vi "相机4图像处理.vi"(6 "生产统计4":T1, 8 "零件型号":string, 9 "工单信息":T2, 10 "自动":bool, 11 "Image Out":T3) -> (0 "生产统计4":T1, 1 "4处理时间":u16, 2 "4结果":bool=TRUE, 3 "Img out":T3(plugin-control))   [LabVIEW 2014]
uses:
  Controls/ProductNum.ctl
  <vilib>/vision/Image Controls.llb/IMAQ Image.ctl
panel:
  in  "显示坐标":cluster{dbl, "Numeric":dbl}[](array[cluster])=[{300.0, "Numeric"=200.0}, {300.0, "Numeric"=400.0}, {300.0, "Numeric"=600.0}, {300.0, "Numeric"=800.0}, {300.0, "Numeric"=1000.0}, {300.0, "Numeric"=1200.0}, {300.0, "Numeric"=1400.0}]
  in  "Img Path":path=path "E:/X-Max总装机3-2019200319/实验图片/4号相机/4.bmp"
  # "%"
  # "%"
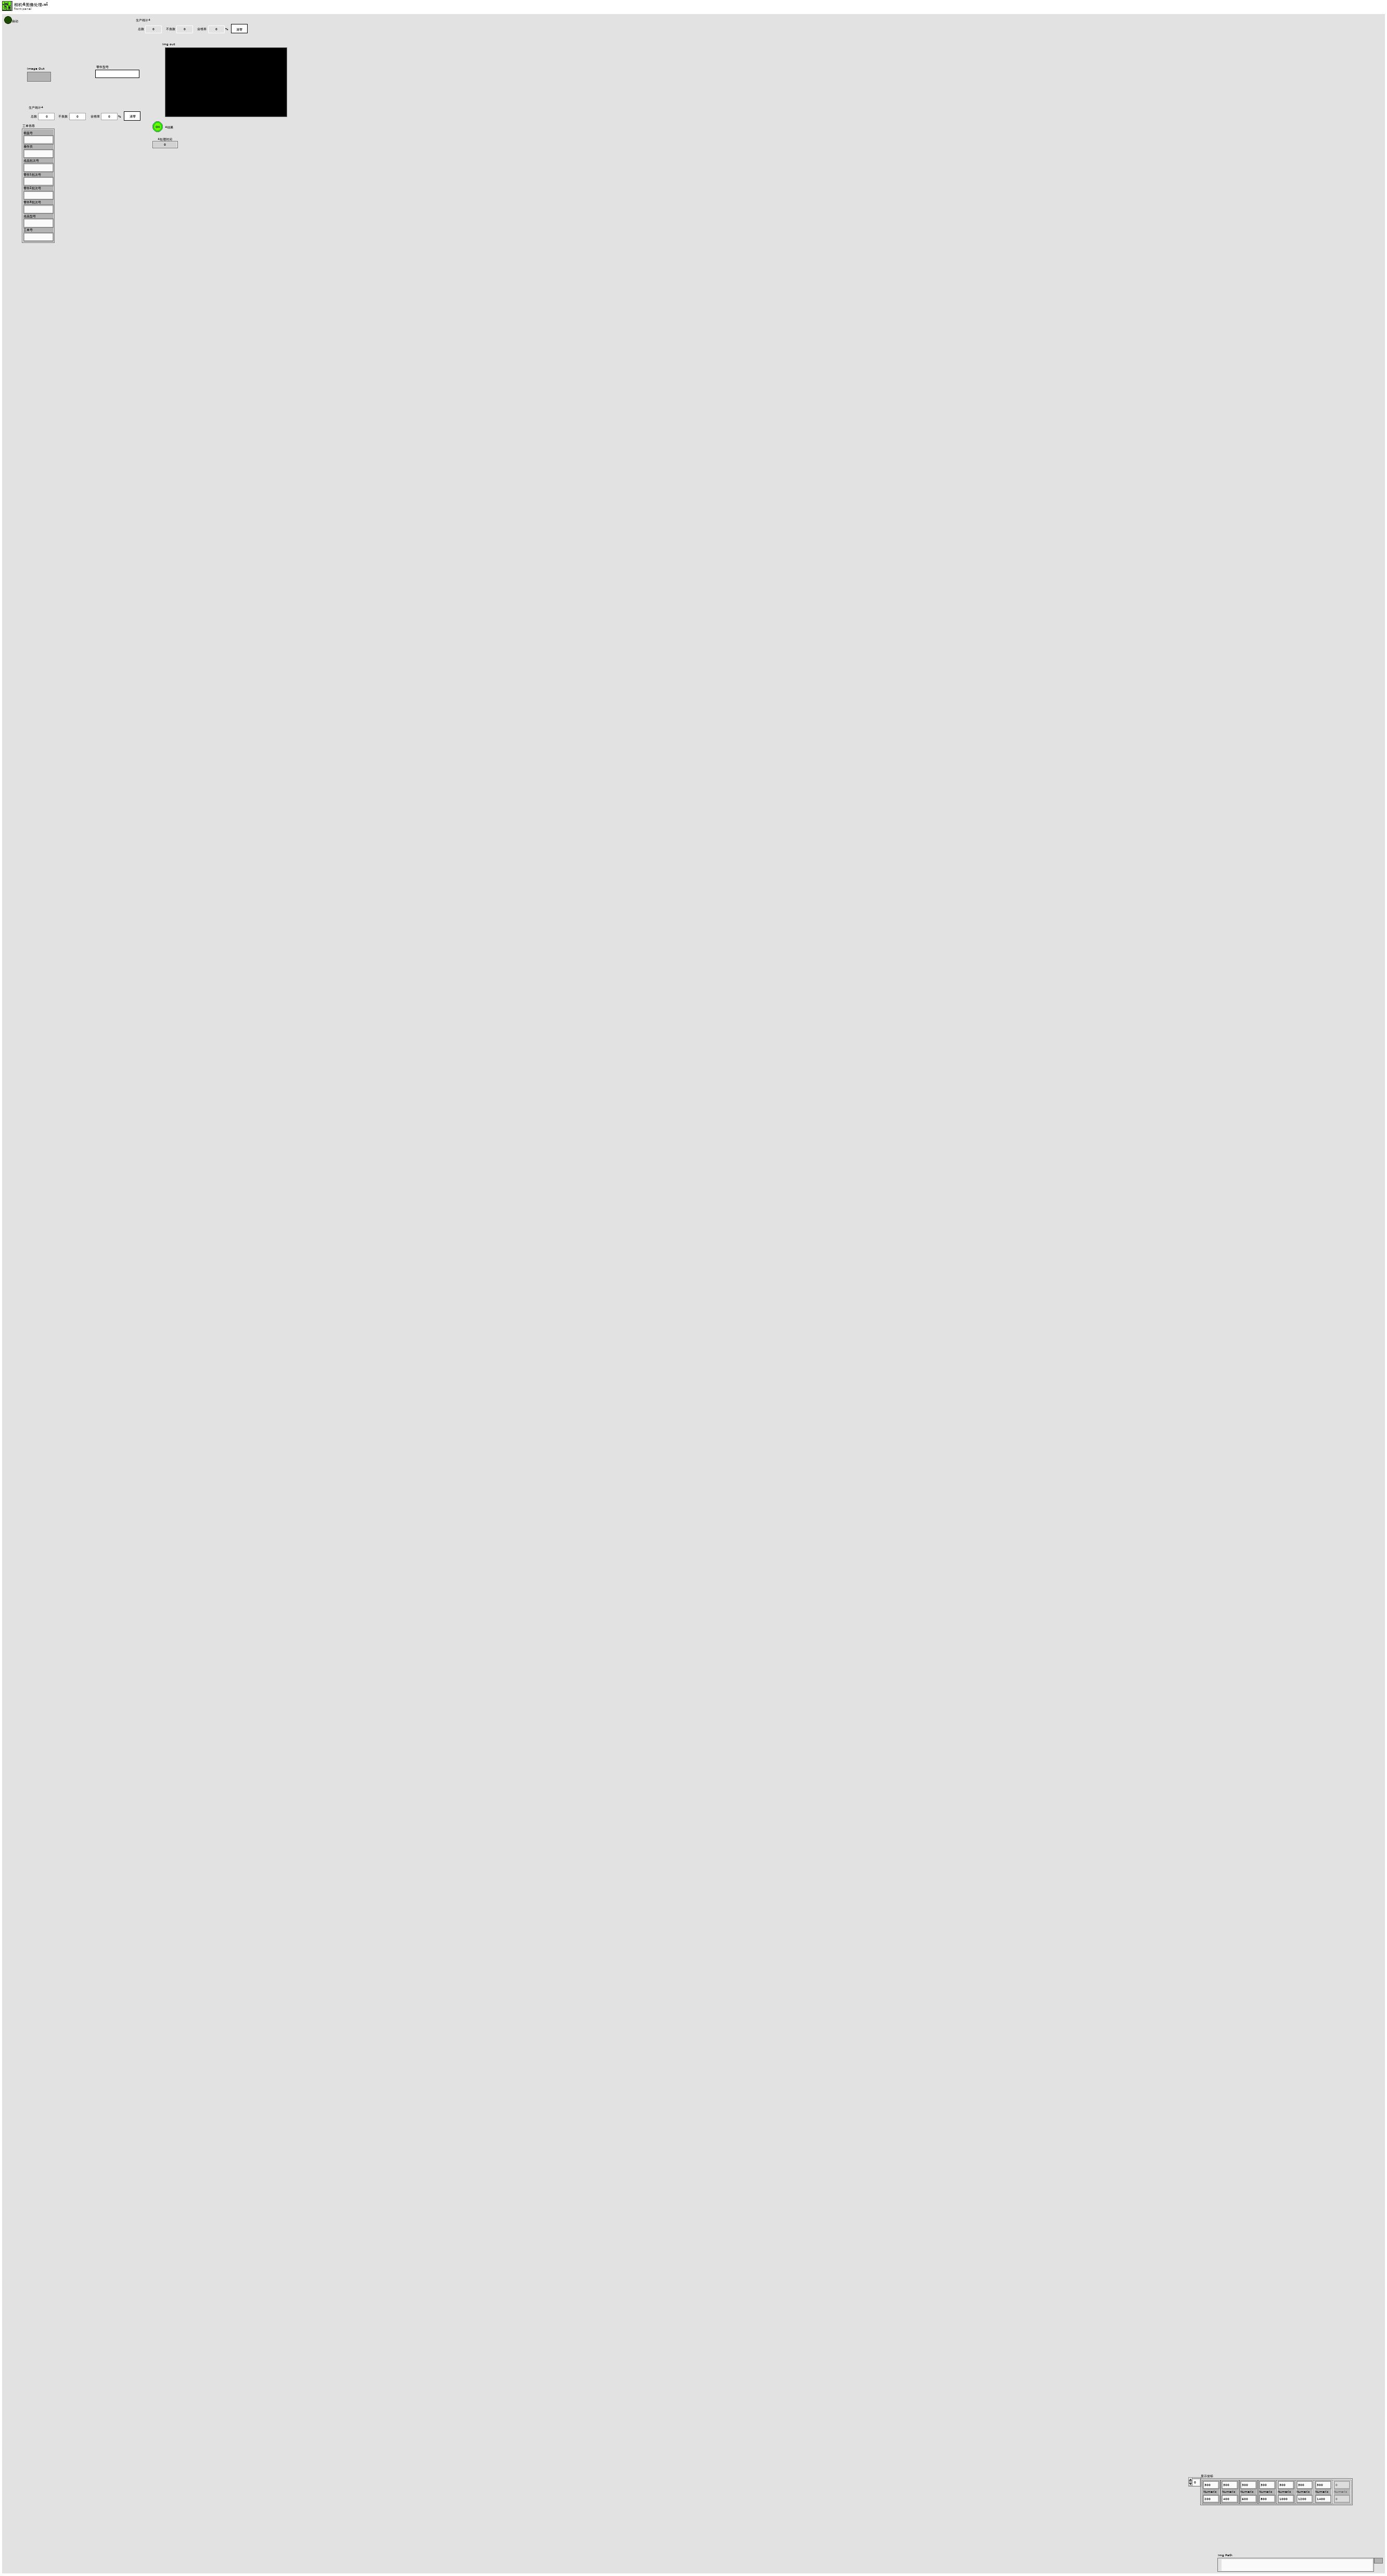
[diagram p1: front panel]
types:
  T1 = typedef "ProductNum.ctl" = cluster{"总数":u64, "不良数":u64, "合格率":dbl, "清零":bool}
  T2 = cluster{"载盘号":string, "操作员":string, "成品批次号":string, "零件1批次号":string, "零件2批次号":string, "零件3批次号":string, "成品型号":string, "工单号":string}
  T3 = typedef "IMAQ Image.ctl" = refnum<image>
  T4 = cluster{"Center (Pixels)":cluster{"X":sgl, "Y":sgl}, "Radius (Pixels)":dbl, "Center (Real-World)":cluster{"X":sgl, "Y":sgl}, "Radius (Real-World)":dbl, "Roundness (Real-World)":dbl, "Average Strength":dbl, "Average SNR (dB)":dbl}
  T5 = typedef "升立德IOAction.ctl" = enum16{"IO卡初始化", "读信号(16bit)", "写信号(16bit)", "写拍照完成信号OFF", "写拍照完成信号ON", "写拍照结果", "GetInfo", "清除目标"}
  T6 = typedef "控件-写数据到PLC Action.ctl" = enum16{"PLC通讯初始化", "PLC通讯初始化2", "读触发信息", "读工单信息", "写工单切换成功", "写入相机1拍照结果", "写入相机2拍照结果", "写入相机3拍照结果", "写入相机4拍照结果", "写入生命信号", "断开连接"}
  T7 = typedef "控件-存档数据和结果.ctl" = cluster{"待写入数据":dbl[], "单个结果":bool[], "总结果":bool, "有效数据":bool}
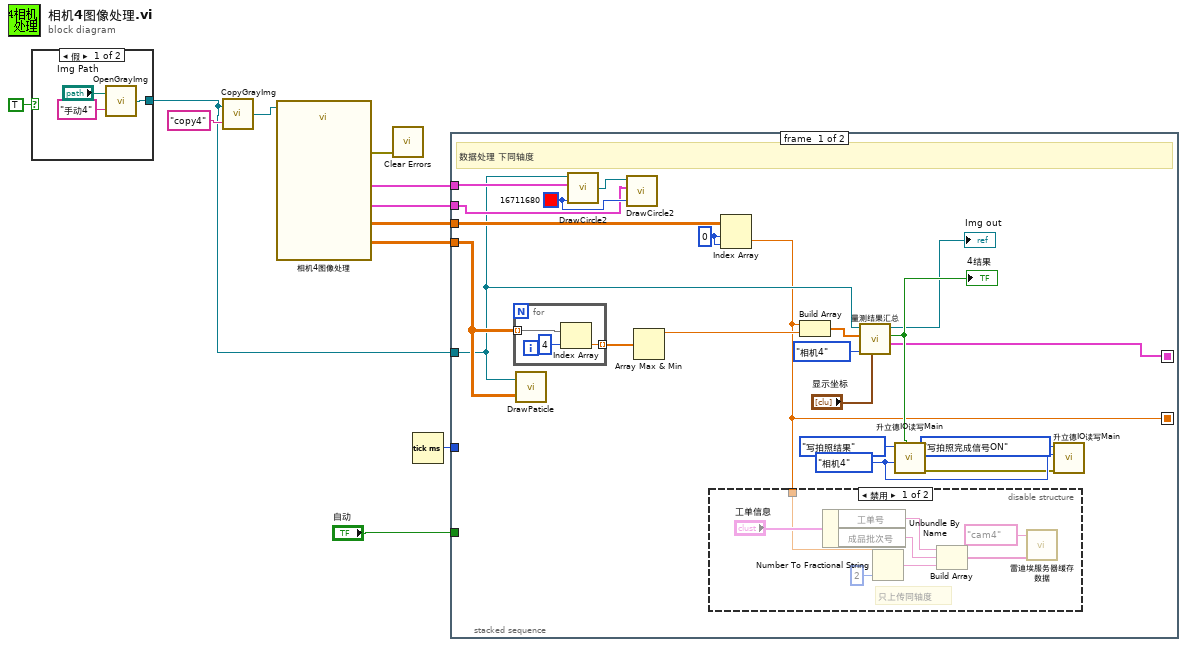
[diagram p0: block diagram]
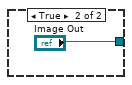
[diagram p2: hidden frame]
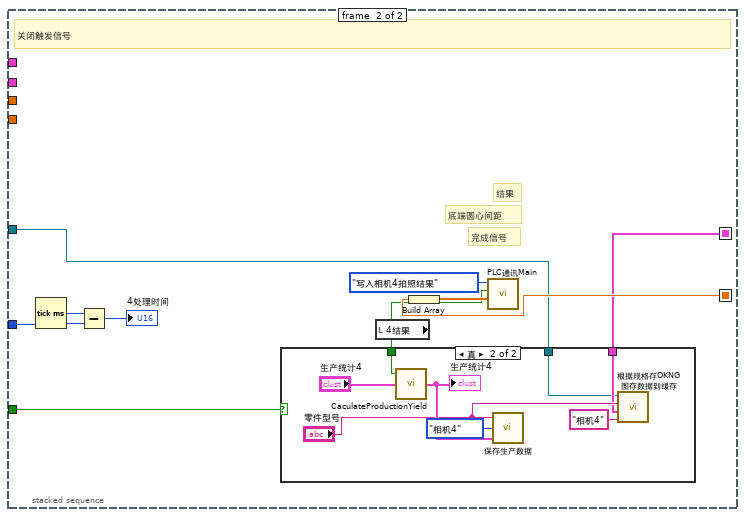
[diagram p4: hidden frame]
diagram:
  n1 = case shown="假" TRUE {
    tunnel: [w14 "Image Out"] -> w1
    frame False {
      n2 = call "OpenGrayImg.vi"("Image Name"="手动4", "Img Path"="Img Path") -> ("Image Out"=w14:T3)
    }
    frame True {
    }
  }
  n3 = call "CopyGrayImg.vi"("Image Name"="copy4", "Image In"=w1) -> ("Image Out"=w11:T3)
  n4 = call "相机4图像处理"("Image In"=w11) -> ("Fitted Circle (内导体检测)"=w7:T4, "Particle Measurements (Pixels) (Particle Analysis 1)"=w9:dbl[][], "Fitted Circle (外导体检测)"=w6:T4, "Caliper Results (Caliper 1)"=w8:sgl[][], "error out"=w10:errorcluster)  [unwired: 21 in, 1 out]
  n5 = call <vilib>:"Clear Errors.vi"("error in (no error)"=w10) -> ()  [unwired: 5 in, 2 out]
  n6 = Tick Count (ms)() -> (millisecond timer value=w5:u32)
  n7 = stacked-sequence {
    seq-local: [w16 _] -> [_ w52]
    seq-local: [w21 _] -> [_ w49]
    tunnel: w5 -> [_ w57]
    tunnel: w1 -> [w20 w48]
    tunnel: w6 -> [w24 _]
    tunnel: w7 -> [w23 _]
    tunnel: w8 -> [w35 _]
    tunnel: w9 -> [w31 _]
    tunnel: "自动" -> [_ w50]
    frame #0 {
      w25 = u32 16711680 ("Color")
      w30 = enum16{"相机1", "相机2", "相机3", "相机4"}."相机4" ("选择相机")
      w36 = 0 ("索引 (行)")
      # "数据处理 下同轴度"
      n8 = for {
        tunnel: w31 -> [w47] mode=indexing
        tunnel: [w45] -> w34 mode=indexing
        n9 = Index Array(array=w47, index=4 ("索引")) -> (element=w45:dbl)
      }
      n10 = call "DrawPaticle.vi"("Particle Measurements (Pixels) (左引脚)"=w31, "引用句柄输入"=w20) -> ()  [unwired: 1 out]
      n11 = call "DrawCircle2.vi"("Color"=w25, "Fitted Circle (左圆)"=w24, "Img in"=w20) -> ("Img out"=w26:T3)  [unwired: 1 in]
      n12 = call "DrawCircle2.vi"("Color"=w25, "Fitted Circle (左圆)"=w23, "Img in"=w26) -> ()  [unwired: 1 in, 1 out]
      n13 = Array Max & Min(array=w34) -> (max value=w33:dbl)  [unwired: 3 out]
      n14 = Index Array(array=w35, index (row)=w36, index (col)=w36) -> (element=w16:sgl)
      n15 = disable-structure shown="禁用" {
        disable-tunnel: w16 -> [w37 _]
        frame Disabled {
          # "只上传同轴度"
          n16 = Unbundle By Name("工单信息") -> ("工单号"=w42:string, "成品批次号"=w44:string)
          n17 = Number To Fractional String(number=w37, precision (6)=i16 2 ("精度(6)")) -> (F-format string=w41:string)  [unwired: 2 in]
          n18 = Build Array(w42, w44, w41) -> (w43:string[])
          n19 = call "雷迪埃服务器缓存数据.vi"("cam3数据"=w43, "缓存选择器"="cam4") -> ()  [unwired: 10 in]
        }
        frame Enabled {
        }
      }
      n20 = Build Array(w16, w33) -> (w32:dbl[])
      n21 = call "量测结果汇总.vi"("显示坐标"="显示坐标", "选项"=enum16{"相机1", "相机2", "相机3", "相机4"}."相机4", "量测数据1维"=w32, "Img in"=w20) -> ("存档数据"=w21:T7, "结果"=w22:bool, "ImgOut"=→"Img out":T3)  [unwired: 3 in]
      "4结果" <- w22
      n22 = call "升立德IO读写Main.vi"(7:w22, "选择相机"=w30, "选项"=升立德IOAction."写拍照结果") -> ("error out"=w29:errorcluster)  [unwired: 4 in, 4 out]
      n23 = call "升立德IO读写Main.vi"("error in"=w29, "选择相机"=w30, "选项"=升立德IOAction."写拍照完成信号ON") -> ()  [unwired: 4 in, 5 out]
    }
    frame #1 {
      # "完成信号"
      # "底端圆心间距"
      # "结果"
      # "关闭触发信号"
      n24 = Tick Count (ms)() -> (millisecond timer value=w56:u32)
      n25 = Subtract(x=w56, y=w57) -> (x-y=→"4处理时间":u32)
      n26 = local read "4结果"() -> (w51:bool)
      n27 = case shown="真" w50 {
        tunnel: w51 -> [_ w64]
        tunnel: w49 -> [_ w59]
        tunnel: w48 -> [_ w58]
        frame False {
        }
        frame True {
          n28 = call "CaculateProductionYield.vi"("生产统计"="生产统计4", "Result(in)"=w64) -> ("良率统计out"=w63:T1)  [unwired: 1 in]
          "生产统计4" <- w63
          n29 = call "保存生产数据.vi"("良率统计"=w63, "选择拍照内容"=enum16{"相机1", "相机2", "相机3", "相机4"}."相机4" ("选择相机"), "产品型号"="零件型号") -> ()
          n30 = call "根据规格存OKNG图存数据到缓存.vi"("选择相机字符串"="相机4", "存档数据和结果"=w59, "当前零件型号"="零件型号", "Img输入"=w58) -> ()  [unwired: 8 in]
        }
      }
      n31 = Build Array(w52) -> (w53:sgl[])
      n32 = call "PLC通讯Main.vi"("写入数据"=w53, "拍照结果"=w51, "写入数据Action"=控件-写数据到PLC_Action."写入相机4拍照结果") -> ()  [unwired: 4 in, 5 out]
    }
  }
